vi "Stop Core.vi"(10 "final error code":i32, 11 "Universal Card in":refnum<class "Universal Card.lvclass">) -> (3 "Universal Card out":refnum<class "Universal Card.lvclass">)   [LabVIEW 2013, in "Universal Power Meter.lvlib" / "Universal Card.lvclass"]
doc: "(<B>Filename</B>: Actor Framework.lvlib:Actor.lvclass:Stop Core.vi)\n\nDefines what the actor does before it stops. Use the <B>final error code</B> input to determine whether the actor shut down in response to an error.\n\nBy default, this method does nothing. A descendant class may override it to define behavior, such as shutting down any processes the actor initiated in its override of the Actor Core method."
uses:
  Universal Card.lvclass
  Generic Instrument/Generic Card/Generic Card.lvclass/Generic Card.ctl
  <vilib>/ActorFramework/Actor/Actor.lvclass/Actor.ctl
  Generic Instrument/Generic Card/Generic Card.lvclass
  Universal Power Meter class/Universal Power Meter.lvclass
  <vilib>/ActorFramework/Actor/Actor.lvclass
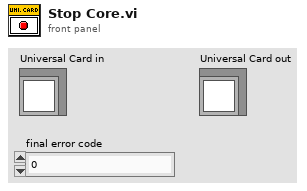
[diagram p1: front panel]
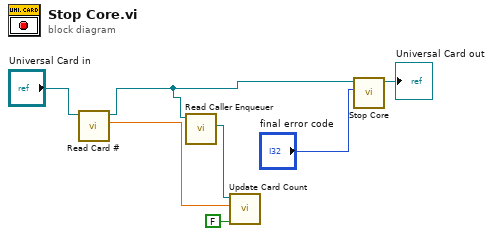
[diagram p0: block diagram]
diagram:
  n1 = call "Read Card #.vi"("Generic Card in"="Universal Card in") -> ("Card #"=w2:dbl, "Generic Card out"=w3:refnum<class "Universal Card.lvclass">)  [unwired: 8 in, 1 out]
  n2 = call <vilib>:"Read Caller Enqueuer.vi"("Actor"=w3) -> ("Caller Enqueuer"=w5:refnum<class "Message Enqueuer.lvclass">)  [unwired: 10 in]
  n3 = call "Update Card Count.vi"("new element/subarray"=FALSE, "# in"=w2, "Message Enqueuer"=w5) -> ()  [unwired: 7 in, 2 out]
  n4 = call-parent "Stop Core.vi"("final error code"="final error code", "Generic Card in"=w3) -> ("Generic Card out"=→"Universal Card out":refnum<class "Universal Card.lvclass">)  [unwired: 9 in]
